vi "Read DATA.vi"(8 "error in (no error)":errorcluster, 11 "Queue in":refnum<class "Queue.lvclass">) -> (0 "error out":errorcluster, 2 "DATA":T1, 3 "Queue out":refnum<class "Queue.lvclass">)   [LabVIEW 2020, in "Data Communication Transmitter.lvlib" / "Queue.lvclass"]
doc: "This VI is used as an API to read data from the queue"
uses:
  Classes/Children/Intra-Application/Children/With Data/Children/Queues/Queue.lvclass
  Classes/Children/Intra-Application/Children/With Data/Children/Queues/Queue.lvclass/Queue.ctl
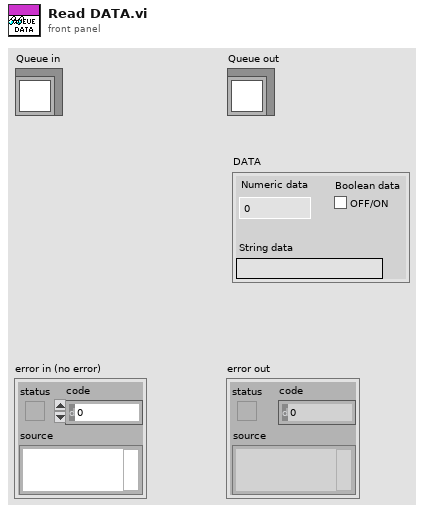
[diagram p1: front panel]
types:
  T1 = cluster{"Numeric data":dbl, "String data":string, "Boolean data":bool}
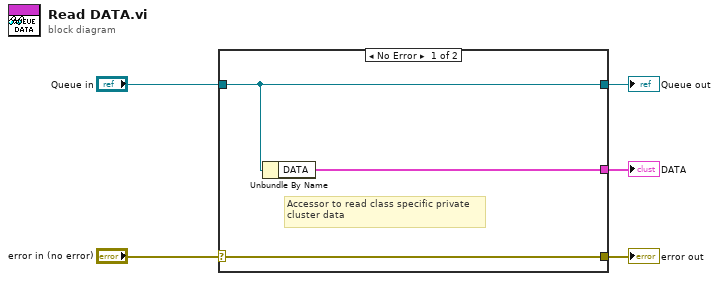
[diagram p0: block diagram]
diagram:
  n1 = case shown="No Error" "error in (no error)" {
    selector: "error in (no error)" -> [w8 w9]
    tunnel: [w8 w9] -> w4
    tunnel: [w7 w10] -> w2
    tunnel: "Queue in" -> [w7 w10]
    tunnel: [w6 _] -> w1
    frame No Error {
      # "Accessor to read class specific private\ncluster data"
      n2 = Unbundle By Name(w7) -> ("DATA"=w6:T1)
    }
    frame Error {
    }
  }
  "error out" <- w4
  "Queue out" <- w2
  "DATA" <- w1
